vi "Bit Unpack.vi"(10 "Num Bits":i32, 11 "Data":u8[](array[numeric])) -> (3 "Unpacked Data":bool[](array[boolean]))   [LabVIEW 2020, in "Device.lvlib"]
uses:
  Device.lvlib
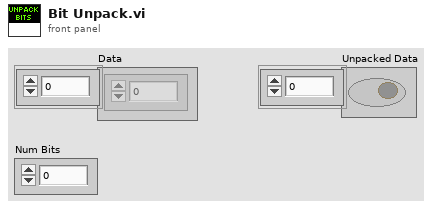
[diagram p1: front panel]
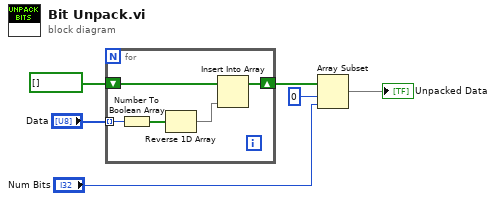
[diagram p0: block diagram]
diagram:
  n1 = for {
    tunnel: "Data" -> [w11] mode=indexing
    shift-right: [w9] -> w3
    shift-left: bool[] [] ("Boolean array") -> [w10]
    n2 = Number To Boolean Array(number=w11) -> (Boolean array=w8:bool[])
    n3 = Reverse 1D Array(array=w8) -> (reversed array=w7:bool[])
    n4 = Insert Into Array(array=w10, new element=w7) -> (w9:bool[])  [unwired: 1 in]
  }
  n5 = Array Subset(array=w3, index=0, length="Num Bits") -> (→"Unpacked Data":bool[])
